vi "WriteData.vi"(8 "Error In":errorcluster, 10 "Data":string, 11 "reference in":refnum<class "CompressionDecorator.lvclass">) -> (0 "Error Out":errorcluster, 3 "reference in":refnum<class "CompressionDecorator.lvclass">)   [LabVIEW 2020, in "CompressionDecorator.lvclass"]
uses:
  CompressionDecorator.lvclass
  DataSourceDecorator_class/DataSourceDecorator.lvclass
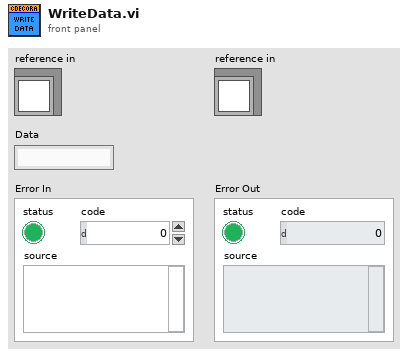
[diagram p1: front panel]
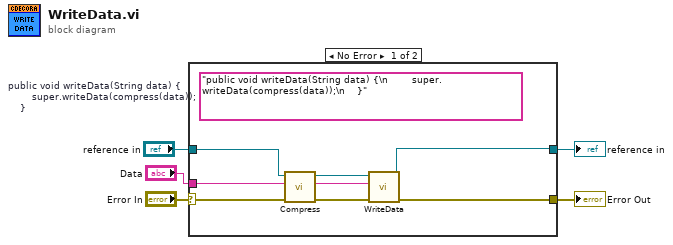
[diagram p0: block diagram]
diagram:
  n1 = case shown="No Error" "Error In" {
    selector: "Error In" -> [w13 w15]
    tunnel: [w12 w15] -> w4
    tunnel: [w6 w14] -> w2
    tunnel: "reference in" -> [w10 w14]
    tunnel: "Data" -> [w7 _]
    frame No Error {
      (unwired) "public void writeData(String data) {\n        super.writeData(compress(data));\n    }"  # public void writeData(String data) {         super.writeData(compress(data));     }
      n2 = call "Compress.vi"("Error In"=w13, "StringData"=w7, "reference in"=w10) -> ("Error Out"=w11:errorcluster, "Return(STRING)"=w8:string, "reference in"=w9:refnum<class "CompressionDecorator.lvclass">)  [unwired: 6 in]
      n3 = call-parent "WriteData.vi"("Error In"=w11, "Data"=w8, "reference in"=w9) -> ("Error Out"=w12:errorcluster, "reference out"=w6:refnum<class "CompressionDecorator.lvclass">)  [unwired: 7 in]
    }
    frame Error {
    }
  }
  "Error Out" <- w4
  "reference in" <- w2
